vi "WS1050 OFFSET CAL updated.vi"(8 "error in":errorcluster, 10 "OFFSET CAL":bool=TRUE) -> (0 "error out":errorcluster)   [LabVIEW 2012]
uses:
  WS_VCAP Driver 029/Source/WSVCAP Shell/Type Defs/WSVCAP SHL I2C DUT Mask Mode Enum.ctl
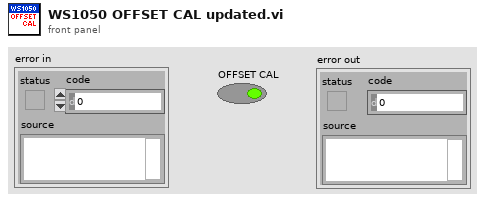
[diagram p1: front panel]
types:
  T1 = typedef "WSVCAP SHL I2C DUT Mask Mode Enum.ctl" = enum16{"Custom", "C1", "C2", "C3", "All"}
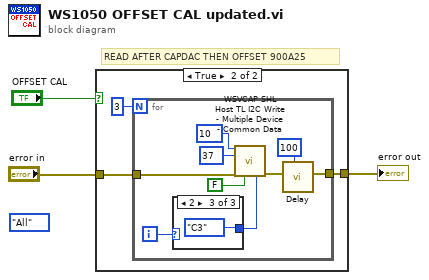
[diagram p0: block diagram]
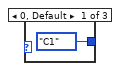
[diagram p3: hidden frame]
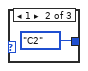
[diagram p4: hidden frame]
diagram:
  (unwired) WSVCAP_SHL_I2C_DUT_Mask_Mode_Enum."All" ("DUT Mask Mode (All)")
  # "READ AFTER CAPDAC THEN OFFSET 900A25"
  n1 = case shown="True" "OFFSET CAL" {
    tunnel: "error in" -> [w4 w7]
    tunnel: [w4 w6] -> w3
    frame False {
    }
    frame True {
      n2 = for {
        N: 3 -> [_]
        tunnel: w7 -> [w16]
        tunnel: [w10] -> w6
        i -> [w12]
        n3 = case shown="2" w12 {
          tunnel: [WSVCAP_SHL_I2C_DUT_Mask_Mode_Enum."C1" ("DUT Mask Mode (All)") WSVCAP_SHL_I2C_DUT_Mask_Mode_Enum."C2" ("DUT Mask Mode (All)") WSVCAP_SHL_I2C_DUT_Mask_Mode_Enum."C3" ("DUT Mask Mode (All)")] -> w11
          frame 0, Default {
          }
          frame 1 {
          }
          frame 2 {
          }
        }
        n4 = call "WSVCAP SHL Host TL I2C Write - Multiple Device - Common Data.vi"("Sub Address"=u8 10, "Data Out [U8]"=u8 37 ("Sub Address"), "error in"=w16, "Log (T)"=FALSE, "DUT Mask Mode (All)"=w11) -> ("error out"=w9:errorcluster)  [unwired: 10 in]
        n5 = call "Delay.vi"("milliseconds to wait"=u32 100, "error in (no error)"=w9) -> ("error out"=w10:errorcluster)  [unwired: 9 in]
      }
    }
  }
  "error out" <- w3
